vi "getChannel.vi"(6 "channel":T1=1 min=1 max=8 step=1, 8 "error in (no error)":errorcluster, 11 "Inst.Krohn-Hite-7008 in":refnum<class "Inst.Krohn-Hite-7008.lvclass">) -> (0 "error out":errorcluster, 2 "channelProperties":variant, 3 "Inst.Krohn-Hite-7008 out":refnum<class "Inst.Krohn-Hite-7008.lvclass">)   [LabVIEW 2019, in "Inst.KH7008.lvlib" / "Inst.Krohn-Hite-7008.lvclass"]
uses:
  Inst.Krohn-Hite-7008.lvclass
  KH7008/typedefs/channel--numeric.ctl
  <userlib>/LevyLab/Instrument Framework/Instrument Types/Amplifier/Instrument.Amplifier.lvclass
  KH7008/KH7008.lvlib
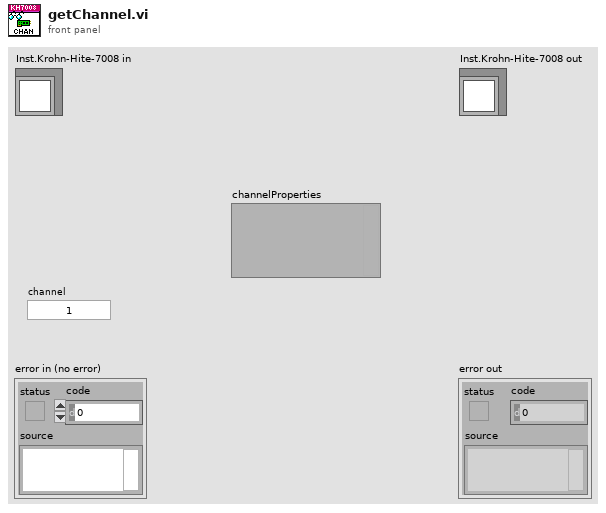
[diagram p1: front panel]
types:
  T1 = typedef "KH7008.lvlib/channel--numeric.ctl" = u16
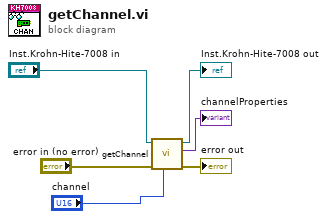
[diagram p0: block diagram]
diagram:
  n1 = call-parent "getChannel.vi"("Channel"="channel", "error in (no error)"="error in (no error)", "Instrument.Amplifier in"="Inst.Krohn-Hite-7008 in") -> ("error out"=→"error out":errorcluster, "channelProperties"=→"channelProperties":variant, "Instrument.Amplifier out"=→"Inst.Krohn-Hite-7008 out":refnum<class "Inst.Krohn-Hite-7008.lvclass">)  [unwired: 6 in]
